vi "R5DOControl_Status.vi"(7 "LabVIEW Web Service Request":refnum<class "Web Request.lvclass">) -> ()   [LabVIEW 2016]
uses:
  <vilib>/wsapi/Web Request.lvclass
  R5Controls/R5DO_Status.ctl
panel:
  out "DO data":T1 {"DO_Manual"."N2 MFC" scale=0.0..500.0; "DO_Manual"."Air MFC" scale=0.0..500.0}
  # "Use the Web Service Request input terminal to call the VIs on the Web Services palette. Do not remove it from the connector pane unless you don't need access to the palette."
  # "Each additional control wired to the connector pane will be available as an input in the URL. To include an indicator in terminal-mode output (the default setting), it must also be wired to the connector pane."
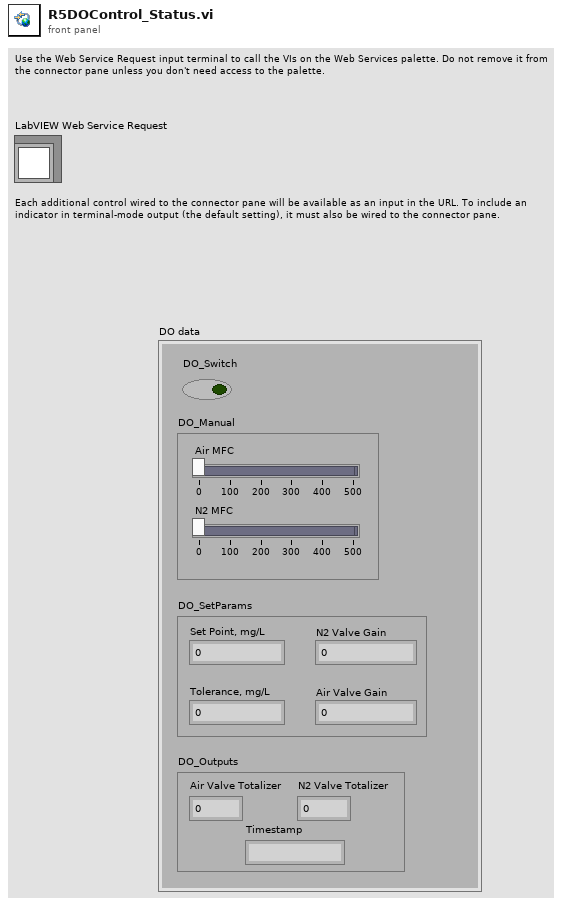
[diagram p1: front panel]
types:
  T1 = typedef "R5DO_Status.ctl" = cluster{"DO_Switch":bool, "DO_Manual":cluster{"Air MFC":dbl, "N2 MFC":dbl}, "DO_Outputs":cluster{"Timestamp":string, "Air Valve Totalizer":dbl, "N2 Valve Totalizer":dbl}, "DO_SetParams":cluster{"Set Point, mg/L":dbl, "Tolerance, mg/L":dbl, "N2 Valve Gain":dbl, "Air Valve Gain":dbl}}
  T2 = cluster{"Set Point, mg/L":dbl, "Tolerance, mg/L":dbl, "N2 Valve Gain":dbl, "Air Valve Gain":dbl}
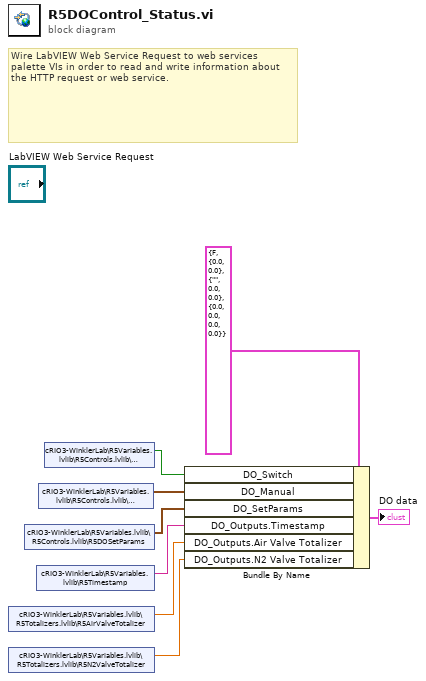
[diagram p0: block diagram]
diagram:
  # "Wire LabVIEW Web Service Request to web services palette VIs in order to read and write information about the HTTP request or web service."
  n1 = shared-variable "cRIO3-WinklerLab\\R5Variables.lvlib\\R5Totalizers.lvlib\\R5AirValveTotalizer"() -> (w7:dbl)  [unwired: 1 in, 1 out]
  n2 = shared-variable "cRIO3-WinklerLab\\R5Variables.lvlib\\R5Totalizers.lvlib\\R5N2ValveTotalizer"() -> (w8:dbl)  [unwired: 1 in, 1 out]
  n3 = shared-variable "cRIO3-WinklerLab\\R5Variables.lvlib\\R5Controls.lvlib\\R5DOSetParams"() -> (w5:T2)  [unwired: 1 in, 1 out]
  n4 = shared-variable "cRIO3-WinklerLab\\R5Variables.lvlib\\R5Timestamp"() -> (w6:string)  [unwired: 1 in, 1 out]
  n5 = shared-variable "cRIO3-WinklerLab\\R5Variables.lvlib\\R5Controls.lvlib\\R5DOManual"() -> (w4:cluster{"Air MFC":dbl, "N2 MFC":dbl})  [unwired: 1 in, 1 out]
  n6 = shared-variable "cRIO3-WinklerLab\\R5Variables.lvlib\\R5Controls.lvlib\\R5DOSwitch"() -> (w3:bool)  [unwired: 1 in, 1 out]
  n7 = Bundle By Name(cluster=T1 {"DO_Switch"=FALSE, "DO_Manual"={"Air MFC"=0.0, "N2 MFC"=0.0}, "DO_Outputs"={"Timestamp"="", "Air Valve Totalizer"=0.0, "N2 Valve Totalizer"=0.0}, "DO_SetParams"={"Set Point, mg/L"=0.0, "Tolerance, mg/L"=0.0, "N2 Valve Gain"=0.0, "Air Valve Gain"=0.0}} ("DOData"), "DO_Switch"=w3, "DO_Manual"=w4, "DO_SetParams"=w5, "DO_Outputs.Timestamp"=w6, "DO_Outputs.Air Valve Totalizer"=w7, "DO_Outputs.N2 Valve Totalizer"=w8) -> (→"DO data":T1)
